vi "Insert Test Loader Cases.vi"(1 "TestTag":string) -> (0 "Cases to Insert":string)   [LabVIEW 2011, in "GraphicalTestRunner.lvlib"]
uses:
  GraphicalTestRunner.lvlib
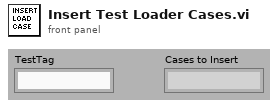
[diagram p1: front panel]
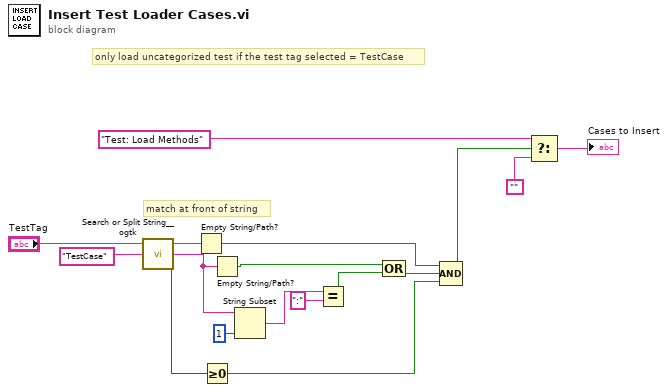
[diagram p0: block diagram]
diagram:
  # "match at front of string"
  # "only load uncategorized test if the test tag selected = TestCase"
  n1 = call <userlib>:"Search or Split String__ogtk.vi"("search string/char (-)"="TestCase" ("y"), "string"="TestTag") -> ("offset after match"=w12:i32, "substring after match"=w3:string, "substring before match"=w14:string)  [unwired: 1 in]
  n2 = Empty String/Path?(string/path=w14) -> (empty?=w15:bool)
  n3 = Greater Or Equal To 0?(x=w12) -> (x >= 0?=w13:bool)
  n4 = Empty String/Path?(string/path=w3) -> (empty?=w8:bool)
  n5 = String Subset(string=w3, length (rest)=1 ("length (rest)")) -> (substring=w2:string)  [unwired: 1 in]
  n6 = Equal?(x=w2, y=":") -> (x = y?=w6:bool)
  n7 = Compound Arithmetic op=OR(w8, w6) -> (w7:bool)
  n8 = Compound Arithmetic op=AND(w15, w7, w13) -> (w1:bool)
  n9 = Select(t="Test: Load Methods" ("y"), s=w1, f="") -> (s? t:f=→"Cases to Insert":string)
